vi "Get Model Information.vi"(8 "error in":errorcluster, 11 "Alicat Device in":refnum<class "Alicat Device.lvclass">) -> (0 "error out":errorcluster, 2 "DataOut":string, 3 "Alicat Device out":refnum<class "Alicat Device.lvclass">)   [LabVIEW 2014, in "Alicat Lib.lvlib" / "Alicat Device.lvclass"]
doc: "Retrieve the model data from the Alicat device using the command <b>X??M*</b> where <b>X</b> is the address of the device. The model data will contain all the information to determine what the device is. This includes the scale, units and model."
uses:
  Alicat Device.lvclass
  Alicat Device.lvclass/Alicat Device.ctl
  reusable/Session APIs/Serial/Public/Asynchronous Write.vi
  reusable/Session APIs/Serial/Public/Asynchronous Read.vi
  reusable/Session APIs/Serial/Serial Session.lvclass
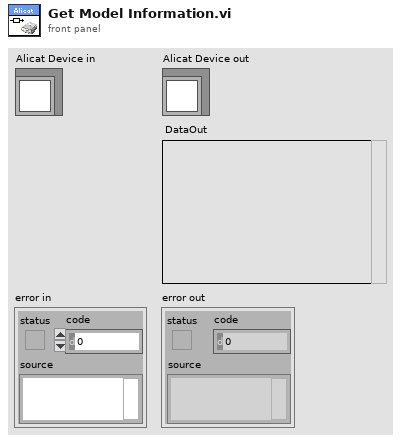
[diagram p1: front panel]
types:
  T1 = typedef "Serial Session.lvclass/Session Handle.ctl" = refnum<data-value>
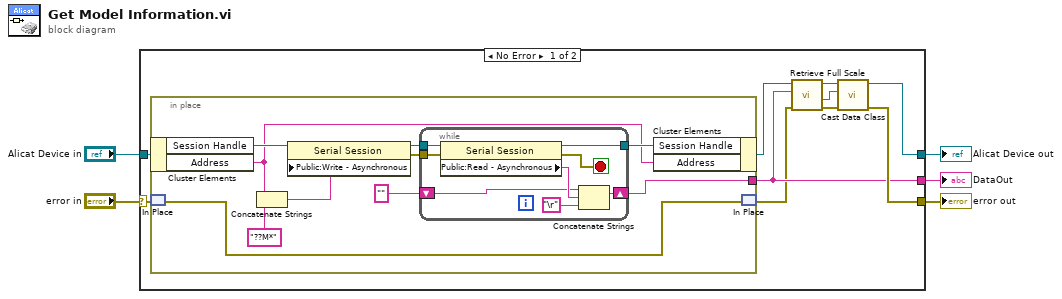
[diagram p0: block diagram]
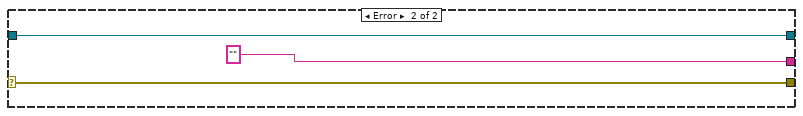
[diagram p2: hidden frame]
diagram:
  n1 = case shown="No Error" "error in" {
    selector: "error in" -> [w14 w36]
    tunnel: "Alicat Device in" -> [w15 w35]
    tunnel: [w13 w36] -> w2
    tunnel: [w12 w35] -> w4
    tunnel: [w11 "" ("DataOut")] -> w1
    frame No Error {
      n2 = in-place {
        in-place-border: [w22] -> w11
        n3 = in-place-cluster #1(w15) -> ("Session Handle"=w24:T1, "Address"=w20:string)
        n4 = in-place-match #2(w14) -> (w21:errorcluster)
        n5 = Concatenate Strings(w20, "??M*" ("string")) -> (w18:string)
        n6 = property class="Serial Session"(reference=w24, "Public:Write - Asynchronous"=w18) -> (reference out=w23:T1, error out=w16:errorcluster)  [unwired: 1 in]
        n7 = while {
          tunnel: w23 -> [w33]
          tunnel: [w28] -> w25
          shift-right: [w30] -> w22
          shift-left: "" -> [w29]
          tunnel: w16 -> [w27]
          stop <- w32 stop-if-true
          n8 = property class="Serial Session"(reference=w33, error in=w27) -> (reference out=w28:T1, error out=w32:errorcluster, "Public:Read - Asynchronous"=w31:string)
          n9 = Concatenate Strings(w29, w31, "\r") -> (w30:string)
        }
        n10 = in-place-cluster #1("Session Handle"=w25, "Address"=w20) -> (w10:refnum<class "Alicat Device.lvclass">)
        n11 = in-place-match #2(w21) -> (w8:errorcluster)
      }
      n12 = call "Retrieve Full Scale.vi"("error in"=w8, "Model Data"=w11, "Alicat Device in"=w10) -> ("error out"=w7:errorcluster, "Type"=w6:string, "Alicat Device out"=w9:refnum<class "Alicat Device.lvclass">)  [unwired: 5 in, 1 out]
      n13 = call "Cast Data Class.vi"("error in"=w7, "Type"=w6, "Alicat Device in"=w9) -> ("error out"=w13:errorcluster, "Alicat Device out"=w12:refnum<class "Alicat Device.lvclass">)  [unwired: 6 in, 1 out]
    }
    frame Error {
    }
  }
  "error out" <- w2
  "Alicat Device out" <- w4
  "DataOut" <- w1
